vi "Teleop.vi"(10 "Match Info":T1={"Autonomous Elapsed Seconds"=0.0, "TeleOp Elapsed Seconds"=0.0, "Disabled Elapsed Seconds"=0.0, "Visited Autonomous"=FALSE, "Visited TeleOp"=FALSE, "Visited Disabled"=FALSE, "Autonomous Settings"={"Autonomous Style"=enum."Independent", "VI Refnum"=refnum}}, 11 "Call Context":T2) -> ()   [LabVIEW 2017]
doc: "This VI is called for each TeleOp packet received from the DS where the robot is not disabled. It is often used to read from the joysticks and update I/O or to update setpoints for timed control loops. It should complete and return within 20 milliseconds or it may miss DS packets."
uses:
  <vilib>/Rock Robotics/WPI/DriverStation/WPI_DriverStationDerivedRobotMode.ctl
  <vilib>/Rock Robotics/WPI/DriverStation/WPI_DriverStationMatch Info.ctl
  <vilib>/Rock Robotics/Network Tables/NT Write Numeric Array.vi
  <vilib>/Rock Robotics/Network Tables/NT Write Boolean Array.vi
  Robot Global Data.vi
  <vilib>/Rock Robotics/Network Tables/NT Read Boolean.vi
  <vilib>/Rock Robotics/Network Tables/NT Read String.vi
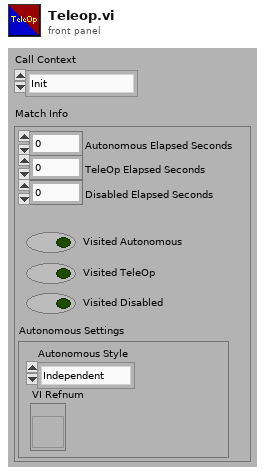
[diagram p1: front panel]
types:
  T1 = typedef "WPI_DriverStationMatch Info.ctl" = cluster{"Autonomous Elapsed Seconds":dbl, "TeleOp Elapsed Seconds":dbl, "Disabled Elapsed Seconds":dbl, "Visited Autonomous":bool, "Visited TeleOp":bool, "Visited Disabled":bool, "Autonomous Settings":cluster{"Autonomous Style":enum16{"Iterative", "Independent"}, "VI Refnum":refnum<vi>}}
  T2 = typedef "WPI_DriverStationDerivedRobotMode.ctl" = enum16{"Init", "Execute", "Stop"}
  T3 = enum16{"1 Xbox Controller", "2 Xbox Controllers"}
  T4 = typedef "TeleopCommands.ctl" = cluster{"Drive Axes":dbl[], "Shooter Forwards":bool, "Shooter Reverse":bool, "Intake Forwards":bool, "Intake Reverse":bool, "Lift Forwards":bool, "Lift Reverse":bool, "Agitator Forwards":bool, "Agitator Reverse":bool, "Left Gear Angle":bool, "Mid Gear Angle":bool, "Right Gear Angle":bool, "Shooter Distance":bool, "Vision Align":bool, "Place Gear":bool, "Command Stop":bool, "Reset Gyro":bool, "Jog Mode?":bool, "Lift Override":bool, "Lift Power":dbl}
  T5 = typedef "WPI_JoystickDevRef.ctl" = cluster{"Device":T6}
  T6 = typedef "WPI_JoystickDeviceEnum.ctl" = enum16{"USB 0", "USB 1", "USB 2", "USB 3", "USB 4", "USB 5"}
  T7 = cluster{"Yaw":dbl, "Roll":dbl, "Pitch":dbl, "Heading":dbl, "Fused Heading":dbl}
  T8 = typedef "WPI_MotorControlDeviceRef.ctl" = cluster{"DeviceStatus":errorcluster, "Type":T9, "PWM":cluster{"PWM Channel":T10, "DeadBand":T11}, "CAN":cluster{"Device Number":u8, "SetOutput VI Ref":variant, "GetOutput VI Ref":variant, "Enable VI Ref":variant, "Disable VI Ref":variant, "Data":variant}, "Invert":bool, "DIO PWM":cluster{"PWM \"Enable\" Channel":T10, "DIOChannel":T12, "PWM Rate":dbl}}
  T9 = typedef "WPI_MotorControlType.ctl" = enum16{"PWM", "CAN", "DIO PWM"}
  T10 = typedef "FPGA_DIOPWMChannel.ctl" = enum8{"PWM 0", "PWM 1", "PWM 2", "PWM 3", "PWM 4", "PWM 5", "PWM 6", "PWM 7", "PWM 8", "PWM 9", "PWM MXP 0", "PWM MXP 1", "PWM MXP 2", "PWM MXP 3", "PWM MXP 4", "PWM MXP 5", "PWM MXP 6", "PWM MXP 7", "PWM MXP 8", "PWM MXP 9", "Invalid"}
  T11 = typedef "WPI_PWMDeadband.ctl" = cluster{"Name":string, "maxPositivePwm":i32, "minPositivePwm":i32, "centerPwm":i32, "maxNegativePwm":i32, "minNegativePwm":i32, "angularRange":u16}
  T12 = typedef "FPGA_DIOChannel.ctl" = enum8{"DIO 0", "DIO 1", "DIO 2", "DIO 3", "DIO 4", "DIO 5", "DIO 6", "DIO 7", "DIO 8", "DIO 9", "DIO MXP 0", "DIO MXP 1", "DIO MXP 2", "DIO MXP 3", "DIO MXP 4", "DIO MXP 5", "DIO MXP 6", "DIO MXP 7", "DIO MXP 8", "DIO MXP 9", "DIO MXP 10", "DIO MXP 11", "DIO MXP 12", "DIO MXP 13", "DIO MXP 14", "DIO MXP 15", "SPI Port CS1", "SPI Port CS2", "SPI Port CS3", "SPI Port MISO", "SPI Port MOSI", "Invalid"}
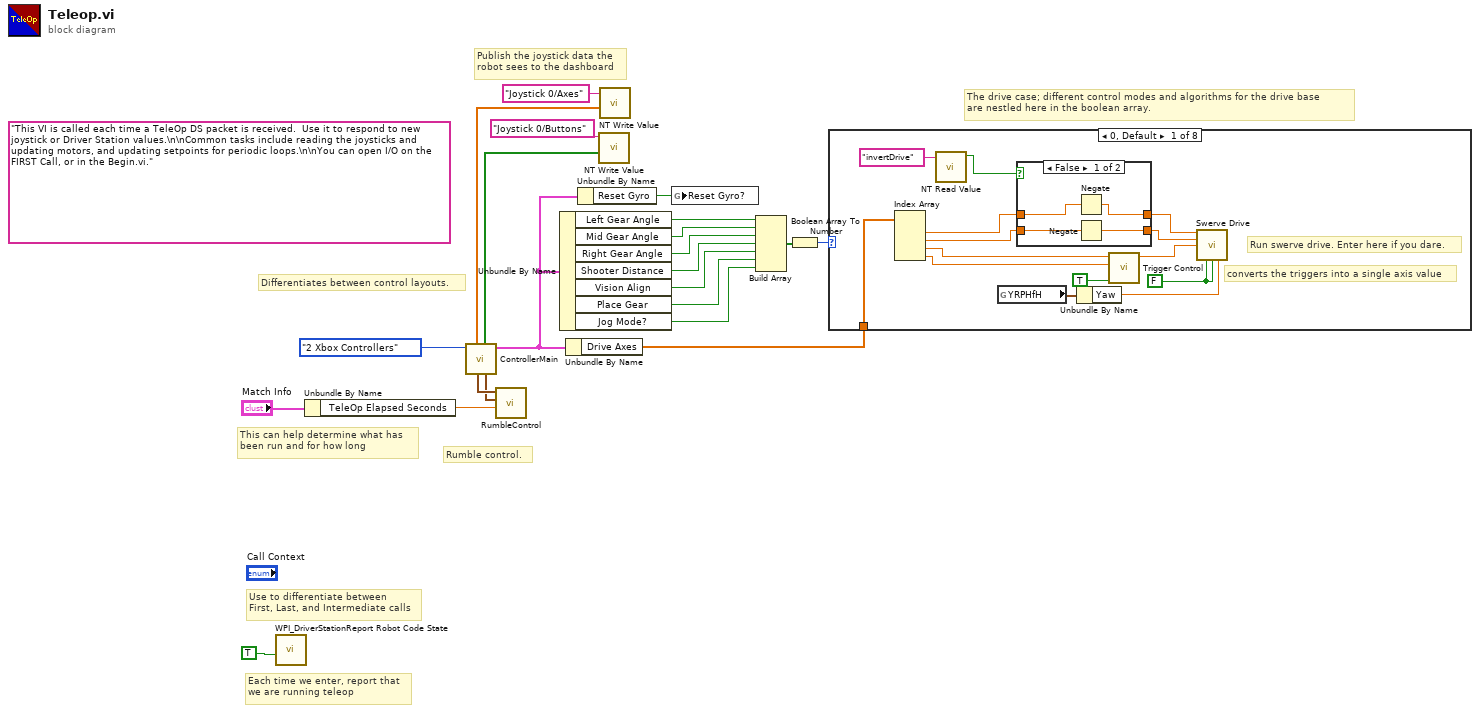
[diagram p0: block diagram]
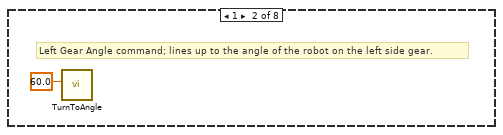
[diagram p3: hidden frame]
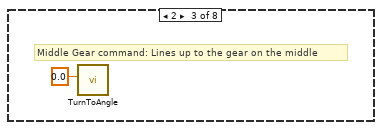
[diagram p4: hidden frame]
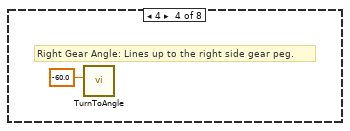
[diagram p5: hidden frame]
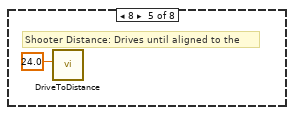
[diagram p6: hidden frame]
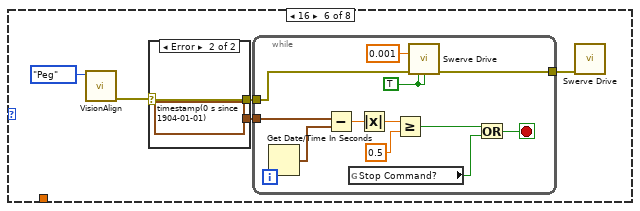
[diagram p7: hidden frame]
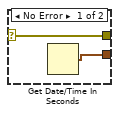
[diagram p8: hidden frame]
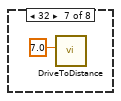
[diagram p9: hidden frame]
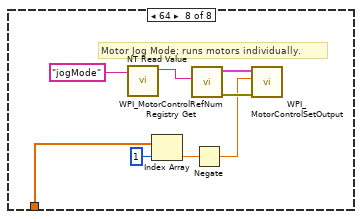
[diagram p10: hidden frame]
diagram:
  (unwired) "This VI is called each time a TeleOp DS packet is received.  Use it to respond to new joystick or Driver Station values.\n\nCommon tasks include reading the joysticks and updating motors, and updating setpoints for periodic loops.\n\nYou can open I/O on the FIRST Call, or in the Begin.vi."
  # "The drive case; different control modes and algorithms for the drive base \nare nestled here in the boolean array."
  # "Rumble control."
  # "Differentiates between control layouts."
  # "Publish the joystick data the\nrobot sees to the dashboard"
  # "Each time we enter, report that\nwe are running teleop"
  # "Use to differentiate between\nFirst, Last, and Intermediate calls"
  # "This can help determine what has\nbeen run and for how long"
  n1 = call <vilib>:"WPI_DriverStationReport Robot Code State.vi"("TeleOp"=TRUE ("Autonomous")) -> ()  [unwired: 10 in, 1 out]
  n2 = Unbundle By Name("Match Info") -> ("TeleOp Elapsed Seconds"=w11:dbl)
  n3 = call "ControllerMain.vi"("Control Mode"=T3."2 Xbox Controllers") -> ("Robot Inputs"=w9:T4, "Joystick1DevRef"=w12:T5, "Stick0 Buttons"=w15:bool[], "Joystick0DevRef"=w13:T5, "Stick0 Axes"=w16:dbl[])  [unwired: 5 in, 1 out]
  n4 = call "RumbleControl.vi"("Teleop Time"=w11, "JoystickDevRef1"=w12, "JoystickDevRef0"=w13) -> ()  [unwired: 8 in, 1 out]
  n5 = Unbundle By Name(w9) -> ("Left Gear Angle"=w8:bool, "Mid Gear Angle"=w7:bool, "Right Gear Angle"=w6:bool, "Shooter Distance"=w5:bool, "Vision Align"=w4:bool, "Place Gear"=w3:bool, "Jog Mode?"=w1:bool)
  n6 = Unbundle By Name(w9) -> ("Drive Axes"=w18:dbl[])
  n7 = Unbundle By Name(w9) -> ("Reset Gyro"=w2:bool)
  n8 = call-poly <vilib>:"NT Write Value.vi"("Boolean Array"=w15, "Name"="Joystick 0/Buttons") -> ()  [unwired: 9 in, 1 out]
  n9 = call-poly <vilib>:"NT Write Value.vi"("Numeric Array"=w16, "Name"="Joystick 0/Axes") -> ()  [unwired: 9 in, 1 out]
  n10 = global write "Robot Global Data.vi" "Reset Gyro?"(w2) -> ()
  n11 = Build Array(w8, w7, w6, w5, w4, w3, w1) -> (w14:bool[])
  n12 = Boolean Array To Number(Boolean array=w14) -> (number=w10:u32)
  n13 = case shown="0, Default" w10 {
    tunnel: w18 -> [w36 _ _ _ _ _ _ w76]
    frame 0, Default {
      w29 = FALSE ("Robot Centric?")
      # "converts the triggers into a single axis value"
      # "Run swerve drive. Enter here if you dare."
      n14 = Index Array(array=w36) -> (element #1=w28:dbl, element #2=w27:dbl, element #3=w35:dbl, element #4=w34:dbl)  [unwired: 4 in]
      n15 = call-poly <vilib>:"NT Read Value.vi"("Name"="invertDrive") -> ("Boolean"=w23:bool)  [unwired: 9 in, 1 out]
      n16 = global read "Robot Global Data.vi" "YRPHfH"() -> (w31:T7)
      n17 = case shown="False" w23 {
        tunnel: w28 -> [w40 w42]
        tunnel: w27 -> [w39 w41]
        tunnel: [w38 w42] -> w26
        tunnel: [w37 w41] -> w25
        frame False {
          n18 = Negate(x=w40) -> (-x=w38:dbl)
          n19 = Negate(x=w39) -> (-x=w37:dbl)
        }
        frame True {
        }
      }
      n20 = Unbundle By Name(w31) -> ("Yaw"=w30:dbl)
      n21 = call "Trigger Control.vi"("Invert?"=TRUE, "Axis 2 In"=w34, "Axis 1 In"=w35) -> ("Axis Out"=w32:dbl)  [unwired: 8 in]
      n22 = call "Swerve Drive.vi"("X"=w26, "Y"=w25, "Z"=w32, "Robot Centric?"=w29, "Autonomous?"=w29, "Yaw"=w30) -> ()  [unwired: 5 in, 5 out]
    }
    frame 1 {
      # "Left Gear Angle command; lines up to the angle of the robot on the left side gear."
      n23 = call "TurnToAngle.vi"("Target Angle"=60.0) -> ()  [unwired: 10 in, 1 out]
    }
    frame 2 {
      # "Middle Gear command: Lines up to the gear on the middle"
      n24 = call "TurnToAngle.vi"("Target Angle"=0.0) -> ()  [unwired: 10 in, 1 out]
    }
    frame 4 {
      # "Right Gear Angle: Lines up to the right side gear peg."
      n25 = call "TurnToAngle.vi"("Target Angle"=-60.0) -> ()  [unwired: 10 in, 1 out]
    }
    frame 8 {
      # "Shooter Distance: Drives until aligned to the"
      n26 = call "DriveToDistance.vi"("Setpoint"=24.0) -> ()  [unwired: 10 in, 1 out]
    }
    frame 16 {
      n27 = call "VisionAlign.vi"("Control Mode"=enum16{"Boiler", "Peg"}."Peg") -> ("Error Out"=w48:errorcluster)  [unwired: 10 in]
      n28 = case shown="Error" w48 {
        selector: w48 -> [w52 w54]
        tunnel: [w53 timestamp(0 s since 1904-01-01) ("seconds since 1Jan1904")] -> w50
        tunnel: [w52 w54] -> w47
        frame No Error {
          n29 = Get Date/Time In Seconds() -> (seconds since 1Jan1904=w53:timestamp)
        }
        frame Error {
        }
      }
      n30 = while {
        tunnel: w50 -> [w67]
        tunnel: [w60] -> w49
        tunnel: w47 -> [w57]
        stop <- w58 stop-if-true
        w62 = TRUE ("Robot Centric?")
        n31 = Get Date/Time In Seconds() -> (seconds since 1Jan1904=w66:timestamp)
        n32 = Subtract(x=w67, y=w66) -> (x-y=w65:dbl)
        n33 = global read "Robot Global Data.vi" "Stop Command?"() -> (w56:bool)
        n34 = Absolute Value(x=w65) -> (abs(x)=w64:dbl)
        n35 = Greater Or Equal?(x=w64, y=0.5) -> (x >= y?=w59:bool)
        n36 = call "Swerve Drive.vi"("Y"=0.001, "Error In"=w57, "Robot Centric?"=w62, "Autonomous?"=w62) -> ("Error Out"=w60:errorcluster)  [unwired: 7 in, 4 out]
        n37 = Or(x=w59, y=w56) -> (x .or. y?=w58:bool)
      }
      n38 = call "Swerve Drive.vi"("Error In"=w49) -> ()  [unwired: 10 in, 5 out]
    }
    frame 32 {
      n39 = call "DriveToDistance.vi"("Setpoint"=7.0) -> ()  [unwired: 10 in, 1 out]
    }
    frame 64 {
      # "Motor Jog Mode; runs motors individually."
      n40 = call-poly <vilib>:"NT Read Value.vi"("Name"="jogMode") -> ("String"=w73:string)  [unwired: 9 in, 1 out]
      n41 = Index Array(array=w76, index=1) -> (element=w74:dbl)
      n42 = call <vilib>:"WPI_MotorControlRefNum Registry Get.vi"("refnum name"=w73) -> ("error out"=w72:errorcluster, "MotorControlDevRef"=w71:T8)  [unwired: 9 in]
      n43 = Negate(x=w74) -> (-x=w70:dbl)
      n44 = call <vilib>:"WPI_MotorControlSetOutput.vi"("error in (no error)"=w72, "Output"=w70, "MotorControlDevRef"=w71) -> ()  [unwired: 6 in, 3 out]
    }
  }
